vi "MotorMoveRelative.vi"(3 "位置":dbl, 4 "axis":i32) -> (1 "返回":i32)   [LabVIEW 2018]
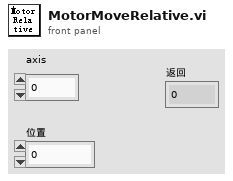
[diagram p1: front panel]
types:
  T1 = cluster{"是否停止":enum16{"解除停止", "停止"}, "发生错误停止运行":enum16{"不停止", "停止"}, "发生错误退出运行":enum16{"不退出", "退出"}, "有效电平":cluster{"脉冲信号有效电平":enum16{"低电平有效", "高电平有效"}, "方向信号有效电平 ":enum16{"低电平有效", "高电平有效"}}, "运行脉宽":i32, "加速度和速度边界":cluster{"加速度最大":i32, "速度最大":i32}, "硬件限位设置":cluster{"正限位使能":enum16{"不使能", "使能"}, "正限位极性":enum16{"低电平有效", "高电平有效"}, "负限位使能 ":enum16{"不使能", "使能"}, "负限位极性 ":enum16{"低电平有效", "高电平有效"}}, "伺服报警":cluster{"伺服报警使能":enum16{"不使能", "使能"}, "伺服报警极性":enum16{"低电平有效", "高电平有效"}}, "电机使能":enum16{"不使能", "使能"}, "输出极性":cluster{"寄存器":u32, " fifo":u32, "Bit":u32, "输出极性控制":enum16{"脉冲+方向", "正负脉冲"}}, "运动模式":enum16{"普通模式", "跟踪模式"}, "加速度 puls/s2":i32, "运动速度":cluster{"峰值速度 puls/s":i32, "起始速度puls/s":i32}, "电机速度归一化常量":dbl, "编码器":cluster{"编码器计数模式":enum16{"正交模式", "脉冲+方向模式"}, "编码器计数方向":enum16{"B相超前A相", "A相超前B相"}, "编码器使能":enum16{"不使能", "使能"}, "寄存器位置":i32, "fifo":i32, "data":i32}, "搜零参数":cluster{"orgSW零点开关":enum16{"0开关作为0点", "正限位作为0点", "负限位作为0点"}, "搜零方向":enum16{"正方向", "负方向"}, "零点停止方式":enum16{"立即停止", "减速停止"}, "原点信号边沿":enum16{"下降沿", "上升沿"}, "判断原点位置方向":enum16{"正方向移动", "负方向移动"}, " reducer搜零方式":enum16{"没有减速装置", "原点边缘作为减速", "探针开关作为减速"}, "零点位置":dbl, "搜零高速度":dbl, "搜零低速度":dbl, " 是否等待结束":enum16{"不等待", "等待"}, "编码器索引信号极性":enum16{"下降沿有效", "上升沿有效"}}}
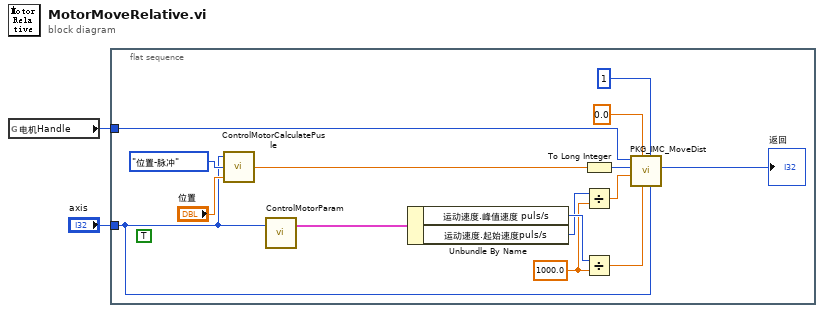
[diagram p0: block diagram]
diagram:
  n1 = global read "参数.vi" "电机Handle"() -> (w2:u32)
  n2 = flat-sequence {
    tunnel: w2 -> [w8]
    tunnel: "axis" -> [w3]
    frame #0 {
      (unwired) TRUE ("状态")
      w11 = 1000.0 ("x")
      n3 = call "ControlMotorCalculatePusle.vi"("数据"="位置", "计算状态"=enum32{"位置-脉冲", "脉冲-位置"}."位置-脉冲", "控制电机"=w3) -> ("dataout"=w16:dbl)  [unwired: 2 in]
      n4 = call "ControlMotorParam.vi"("控制电机"=w3) -> ("轴参数"=w17:T1)  [unwired: 2 in]
      n5 = Unbundle By Name(w17) -> ("运动速度.峰值速度 puls/s"=w15:i32, "运动速度.起始速度puls/s"=w14:i32)
      n6 = To Long Integer(number=w16) -> (32bit integer=w7:i32)
      n7 = Divide(x=w14, y=w11) -> (x/y=w6:dbl)
      n8 = Divide(x=w15, y=w11) -> (x/y=w5:dbl)
      n9 = call "PKG_IMC_MoveDist.vi"("axis"=w3, "wait"=1, "tgvel"=w5, "endvel"=0.0, "startvel"=w6, "dist"=w7, "handle"=w8) -> ("function return"=→"返回":i32)  [unwired: 3 in, 1 out]
    }
  }
